vi "POLARIS two Cameras.vi"() -> ()   [LabVIEW 2009]
uses:
  <vilib>/userDefined/High Color/IMAQdx.ctl
  XDisplay/POLARIS IMAQ Display.xctl
  IMAQdx Cam/IMAQdx Cam.lvclass
  Analyze Classes/Analyze Fluence/Analyze Fluence.lvclass
  XDisplay/Properties/ImageSource.ctl
  Utility/POLARIS Vision utility.lvlib
panel:
  out "error save settings 2":errorcluster
  in  "Camera Name 2":T1="A5-InNF"
  out "POLARIS IMAQ Display 2":cluster{"Image":T2}(xcontrol)
  in  "Energy [J]":dbl
  out "error save settings":errorcluster
  in  "Config Dir":path=path "D:/Test XDisplay images"
  in  "Prefix":string
  in  "WorkDir":path=path "D:/Test XDisplay images"
  out "POLARIS IMAQ Display":cluster{"Image":T2}(xcontrol)
  in  "stop":bool
  in  "Camera Name":T1="JustageCam"
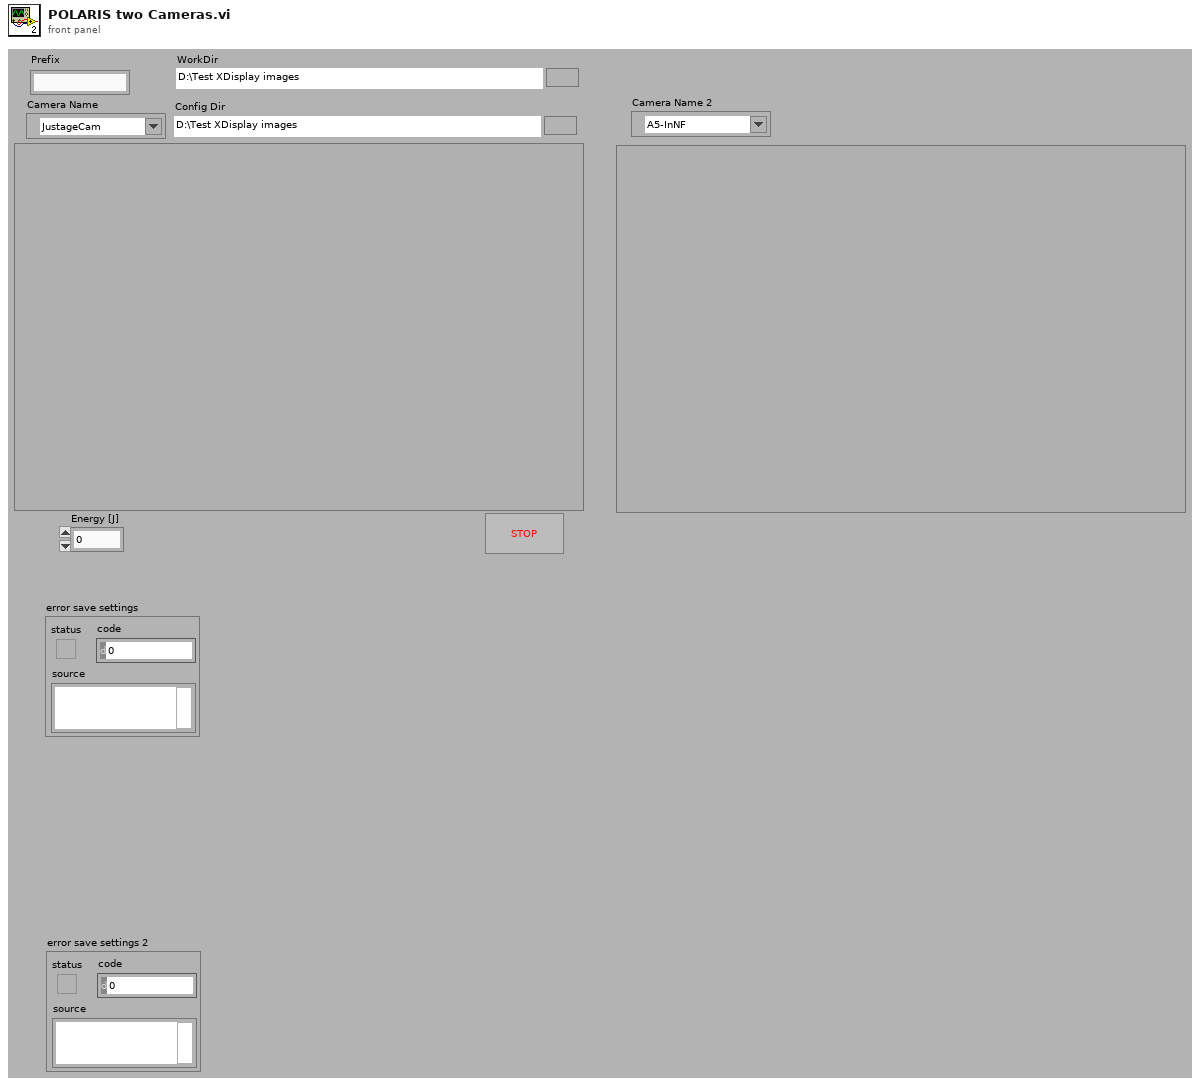
[diagram p1: front panel]
types:
  T1 = typedef "IMAQdx.ctl" = refnum<k21>
  T2 = typedef "IMAQ Image.ctl" = refnum<image>
  T3 = typedef "Image Type" = u32
  T4 = typedef "POLARIS IMAQ Display.xctl/ImageSource.ctl" = enum16{"Camera", "File"}
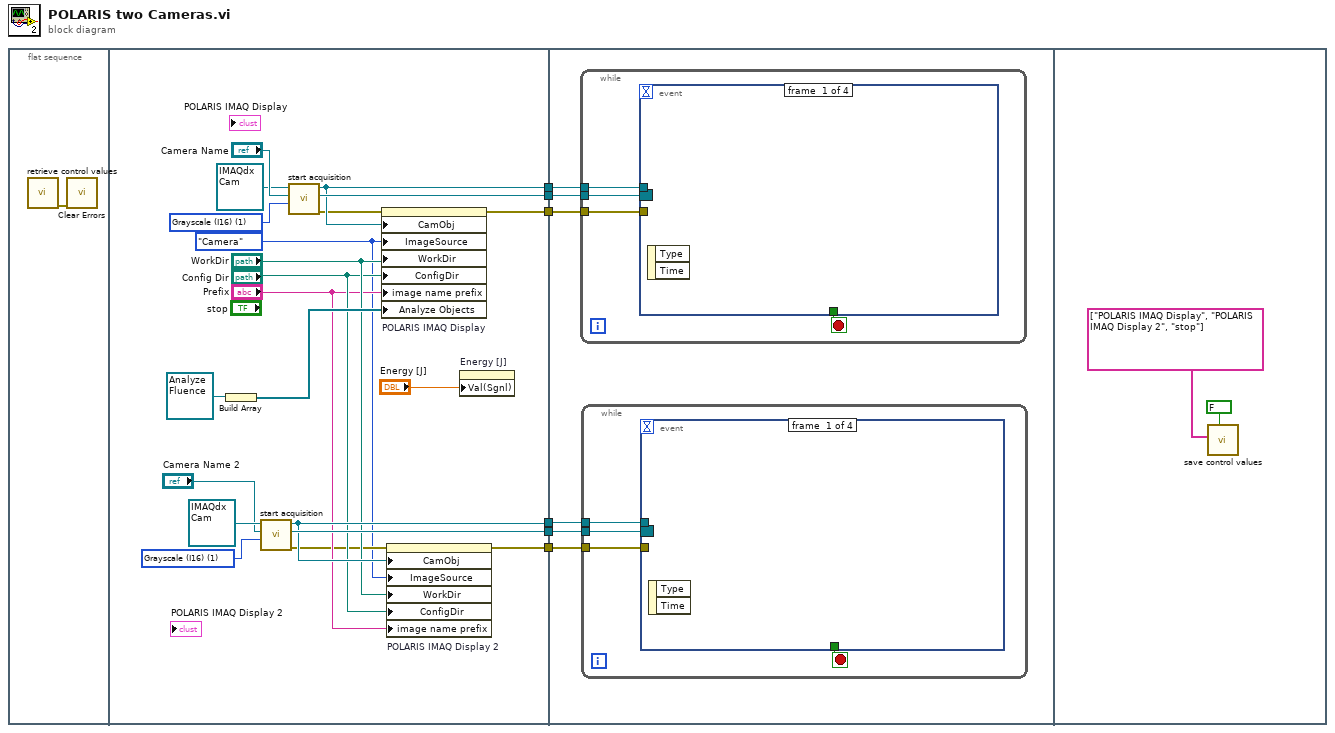
[diagram p0: block diagram]
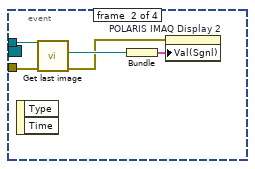
[diagram p2: hidden frame]
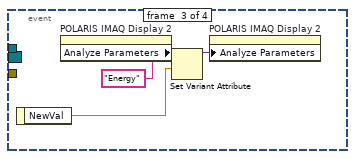
[diagram p3: hidden frame]
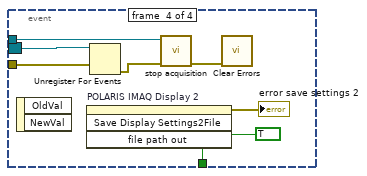
[diagram p4: hidden frame]
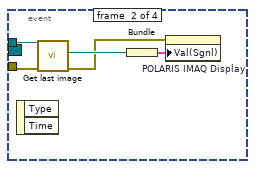
[diagram p5: hidden frame]
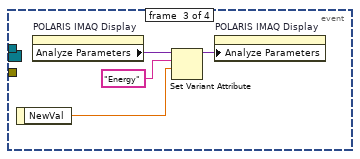
[diagram p6: hidden frame]
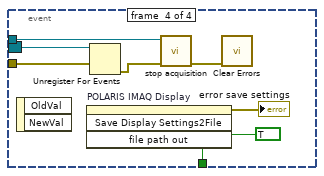
[diagram p7: hidden frame]
diagram:
  n1 = flat-sequence {
    tunnel: [w27] -> w6
    tunnel: [w25] -> w5
    tunnel: [w23] -> w4
    tunnel: [w15] -> w3
    tunnel: [w14] -> w2
    tunnel: [w10] -> w1
    tunnel: w6 -> [w33]
    tunnel: w5 -> [w34]
    tunnel: w4 -> [w32]
    tunnel: w3 -> [w31]
    tunnel: w2 -> [w30]
    tunnel: w1 -> [w29]
    frame #0 {
      n2 = call "retrieve control values.vi"() -> ("error out"=w7:errorcluster)  [unwired: 10 in, 1 out]
      n3 = call <vilib>:"Clear Errors.vi"("error in (no error)"=w7) -> ()  [unwired: 6 in, 1 out]
    }
    frame #1 {
      w18 = T3 1 items=["Grayscale (U8)", "Grayscale (I16)", "Grayscale (SGL)", "Complex (CSG)", "RGB (U32)", "HSL (U32)", "RGB (U64)", "Grayscale (U16)"] ("Image Type")
      w22 = T3 1 items=["Grayscale (U8)", "Grayscale (I16)", "Grayscale (SGL)", "Complex (CSG)", "RGB (U32)", "HSL (U32)", "RGB (U64)", "Grayscale (U16)"] ("Image Type")
      w8 = ImageSource."Camera" ("ImageSource")
      n4 = Build Array(refnum<class "Analyze Fluence.lvclass"> refnum ("Analyze Fluence.lvclass")) -> (w20:refnum<class "Analyze Fluence.lvclass">[])
      n5 = call-dynamic "start acquisition.vi"("Image Type"=w18, "Camera Name"="Camera Name 2", "IMAQdx Cam in"=refnum<class "IMAQdx Cam.lvclass"> refnum ("IMAQdx Cam.lvclass")) -> ("error out"=w9:errorcluster, "Event Registration Refnum"=w15:refnum<event-registration>, "IMAQdx Cam out"=w14:refnum<class "IMAQdx Cam.lvclass">)  [unwired: 6 in]
      n6 = call-dynamic "start acquisition.vi"("Image Type"=w22, "Camera Name"="Camera Name", "IMAQdx Cam in"=refnum<class "IMAQdx Cam.lvclass"> refnum ("IMAQdx Cam.lvclass")) -> ("error out"=w24:errorcluster, "Event Registration Refnum"=w27:refnum<event-registration>, "IMAQdx Cam out"=w25:refnum<class "IMAQdx Cam.lvclass">)  [unwired: 6 in]
      n7 = property on="POLARIS IMAQ Display" class="POLARIS IMAQ Display (strict)"(error in=w24, "CamObj"=w25, "ImageSource"=w8, "WorkDir"="WorkDir", "ConfigDir"="Config Dir", "image name prefix"="Prefix", "Analyze Objects"=w20) -> (error out=w23:errorcluster)  [unwired: 1 in, 1 out]
      n8 = property on="POLARIS IMAQ Display 2" class="POLARIS IMAQ Display (strict)"(error in=w9, "CamObj"=w14, "ImageSource"=w8, "WorkDir"="WorkDir", "ConfigDir"="Config Dir", "image name prefix"="Prefix") -> (error out=w10:errorcluster)  [unwired: 1 in, 1 out]
      n9 = property on="Energy [J]" class="DigNum (strict)"("Val(Sgnl)"="Energy [J]") -> ()  [unwired: 2 in, 2 out]
    }
    frame #2 {
      n10 = while {
        tunnel: w34 -> [w57]
        tunnel: w33 -> [w56]
        tunnel: w32 -> [w55]
        stop <- w58 stop-if-true
        n11 = event shown="[1] <Session Out>: FrameDone" {
          selector: w56 -> [_ _ _ w71]
          dyn-events: _ -> [_ _ _ _]
          timeout: _ -> [_ _ _ _]
          tunnel: [_ _ _ TRUE] -> w58
          tunnel: w57 -> [_ w63 _ w72]
          tunnel: w55 -> [_ w62 _ w70]
          event #0 {
            n12 = event-data() -> ()  [unwired: 1 in, 2 out]
          }
          event #1 {
            n13 = event-data() -> ()  [unwired: 1 in, 2 out]
            n14 = call-dynamic "Get last image.vi"("error in (no error)"=w62, "IMAQdx Cam in"=w63) -> ("error out"=w60:errorcluster, "Image Out"=w61:T2)  [unwired: 7 in, 1 out]
            n15 = Bundle("Image Out"=w61) -> (w59:cluster{"Image Out":T2})  [unwired: 1 in]
            n16 = property on="POLARIS IMAQ Display" class="POLARIS IMAQ Display (strict)"(error in=w60, "Val(Sgnl)"=w59) -> ()  [unwired: 1 in, 2 out]
          }
          event #2 {
            n17 = event-data() -> ("NewVal"=w64:dbl)  [unwired: 1 in]
            n18 = property on="POLARIS IMAQ Display" class="POLARIS IMAQ Display (strict)"() -> ("Analyze Parameters"=w67:variant)  [unwired: 2 in, 2 out]
            n19 = Set Variant Attribute(Variant=w67, name="Energy", value=w64) -> (Variant out=w65:variant)  [unwired: 1 in, 2 out]
            n20 = property on="POLARIS IMAQ Display" class="POLARIS IMAQ Display (strict)"("Analyze Parameters"=w65) -> ()  [unwired: 2 in, 2 out]
          }
          event #3 {
            n21 = event-data() -> ()  [unwired: 1 in, 2 out]
            n22 = invoke on="POLARIS IMAQ Display" class="POLARIS IMAQ Display (strict)" method="Save Display Settings2File"() -> (error out=→"error save settings":errorcluster)  [unwired: 4 in, 3 out]
            n23 = Unregister For Events(event registration refnum=w71, error in=w70) -> (error out=w73:errorcluster)
            n24 = call-dynamic "stop acquisition.vi"("error in (no error)"=w73, "IMAQdx Cam in"=w72) -> ("error out"=w69:errorcluster)  [unwired: 8 in, 1 out]
            n25 = call <vilib>:"Clear Errors.vi"("error in (no error)"=w69) -> ()  [unwired: 6 in, 1 out]
          }
        }
      }
      n26 = while {
        tunnel: w30 -> [w37]
        tunnel: w31 -> [w36]
        tunnel: w29 -> [w35]
        stop <- w38 stop-if-true
        n27 = event shown="[1] <Session Out>: FrameDone" {
          selector: w36 -> [_ _ _ w51]
          dyn-events: _ -> [_ _ _ _]
          timeout: _ -> [_ _ _ _]
          tunnel: [_ _ _ TRUE] -> w38
          tunnel: w37 -> [_ w43 _ w52]
          tunnel: w35 -> [_ w42 _ w50]
          event #0 {
            n28 = event-data() -> ()  [unwired: 1 in, 2 out]
          }
          event #1 {
            n29 = event-data() -> ()  [unwired: 1 in, 2 out]
            n30 = call-dynamic "Get last image.vi"("error in (no error)"=w42, "IMAQdx Cam in"=w43) -> ("error out"=w40:errorcluster, "Image Out"=w41:T2)  [unwired: 7 in, 1 out]
            n31 = Bundle("Image Out"=w41) -> (w39:cluster{"Image Out":T2})  [unwired: 1 in]
            n32 = property on="POLARIS IMAQ Display 2" class="POLARIS IMAQ Display (strict)"(error in=w40, "Val(Sgnl)"=w39) -> ()  [unwired: 1 in, 2 out]
          }
          event #2 {
            n33 = event-data() -> ("NewVal"=w44:dbl)  [unwired: 1 in]
            n34 = property on="POLARIS IMAQ Display 2" class="POLARIS IMAQ Display (strict)"() -> ("Analyze Parameters"=w47:variant)  [unwired: 2 in, 2 out]
            n35 = Set Variant Attribute(Variant=w47, name="Energy", value=w44) -> (Variant out=w45:variant)  [unwired: 1 in, 2 out]
            n36 = property on="POLARIS IMAQ Display 2" class="POLARIS IMAQ Display (strict)"("Analyze Parameters"=w45) -> ()  [unwired: 2 in, 2 out]
          }
          event #3 {
            n37 = event-data() -> ()  [unwired: 1 in, 2 out]
            n38 = invoke on="POLARIS IMAQ Display 2" class="POLARIS IMAQ Display (strict)" method="Save Display Settings2File"() -> (error out=→"error save settings 2":errorcluster)  [unwired: 4 in, 3 out]
            n39 = Unregister For Events(event registration refnum=w51, error in=w50) -> (error out=w53:errorcluster)
            n40 = call-dynamic "stop acquisition.vi"("error in (no error)"=w53, "IMAQdx Cam in"=w52) -> ("error out"=w49:errorcluster)  [unwired: 8 in, 1 out]
            n41 = call <vilib>:"Clear Errors.vi"("error in (no error)"=w49) -> ()  [unwired: 6 in, 1 out]
          }
        }
      }
    }
    frame #3 {
      n42 = call "save control values.vi"("Append timestamp (true)"=FALSE, "Dont save"=string[] ["POLARIS IMAQ Display", "POLARIS IMAQ Display 2", "stop"]) -> ()  [unwired: 6 in, 2 out]
    }
  }
